vi "Grab Frame.vi"(5 "Live?":bool, 7 "Grab frame?":bool, 8 "error in (no error)":errorcluster, 9 "Rigid Body":T1, 11 "Frame Grabber Data in":T4={"Camera Session"="", "Frame"=refnum, "AVI Refnum"=refnum, "Codecs"=[], "Frame number"=0, "Tracking File Refnum"=refnum, "Tick Count"=0, "Probe Object"=refnum, "Playback Probe Data"=[], "Rigid Body"={"Position"={"x (mm)"=0.0, "y (mm)"=0.0, "z (mm)"=0.0}, "Orientation"={"Pitch (rad)"=0.0, "Yaw (rad)"=0.0, "Roll (rad)"=0.0}, "Quaternion"={"qx"=0.0, "qy"=0.0, "qz"=0.0, "qw"=0.0}, "Tracked?"=FALSE}, "Total no frames playback"=0, "Video FPS"=0.0, "Camera connected?"=FALSE, "Scene"=refnum, "Cropped Frame"=refnum, "Tracker FPS"=0.0, "Crop ROI"=[], "Presentation Values"=[], "Elapsed time (ms)"=0, "Camera frames playback"=0, "Refnums"={"Live Refnum"=refnum, "Record Refnum"=refnum, "Recording Settings Refnum"=refnum, "Playback Refnum"=refnum, "Frame Slider Refnum"=refnum, "Pause Refnum"=refnum, "Home Refnum"=refnum, "Crop Refnum"=refnum, "Clear Crop Refnum"=refnum, "stop refnum"=refnum, "Playback Rate Refnum"=refnum, "Operator Settings Refnums"=refnum, "Presentation Refnum"=refnum, "Gestation Refnum"=refnum, "Connection Settings Refnum"=refnum, "Crop Time Frame Slider Refnum"=refnum, "Cancel Save Refnum"=refnum, "Reverse Playback Refnum"=refnum}, "Dimensions"={"Probe Dimensions"={"Probe Width"=0.0, "Probe Depth"=1.0, "Probe Height"=0.0}, "Room Dimensions"={"Room Width"=0.0, "Room Depth"=0.0, "Room Height"=0.0}}, "Playback Data As Strings"=[], "Cropped Tracking File Refnum"=refnum, "Cropped AVI Refnum"=refnum, "Header"=[], "Total euclidian distance"=0.0}) -> (0 "error out":errorcluster, 1 "Elapsed time (ms)":u32, 2 "Frame":T6, 3 "Frame Grabber Data out":T4={"Camera Session"="", "Frame"=refnum, "AVI Refnum"=refnum, "Codecs"=[], "Frame number"=0, "Tracking File Refnum"=refnum, "Tick Count"=0, "Probe Object"=refnum, "Playback Probe Data"=[], "Rigid Body"={"Position"={"x (mm)"=0.0, "y (mm)"=0.0, "z (mm)"=0.0}, "Orientation"={"Pitch (rad)"=0.0, "Yaw (rad)"=0.0, "Roll (rad)"=0.0}, "Quaternion"={"qx"=0.0, "qy"=0.0, "qz"=0.0, "qw"=0.0}, "Tracked?"=FALSE}, "Total no frames playback"=0, "Video FPS"=0.0, "Camera connected?"=FALSE, "Scene"=refnum, "Cropped Frame"=refnum, "Tracker FPS"=0.0, "Crop ROI"=[], "Presentation Values"=[], "Elapsed time (ms)"=0, "Camera frames playback"=0, "Refnums"={"Live Refnum"=refnum, "Record Refnum"=refnum, "Recording Settings Refnum"=refnum, "Playback Refnum"=refnum, "Frame Slider Refnum"=refnum, "Pause Refnum"=refnum, "Home Refnum"=refnum, "Crop Refnum"=refnum, "Clear Crop Refnum"=refnum, "stop refnum"=refnum, "Playback Rate Refnum"=refnum, "Operator Settings Refnums"=refnum, "Presentation Refnum"=refnum, "Gestation Refnum"=refnum, "Connection Settings Refnum"=refnum, "Crop Time Frame Slider Refnum"=refnum, "Cancel Save Refnum"=refnum, "Reverse Playback Refnum"=refnum}, "Dimensions"={"Probe Dimensions"={"Probe Width"=0.0, "Probe Depth"=1.0, "Probe Height"=0.0}, "Room Dimensions"={"Room Width"=0.0, "Room Depth"=0.0, "Room Height"=0.0}}, "Playback Data As Strings"=[], "Cropped Tracking File Refnum"=refnum, "Cropped AVI Refnum"=refnum, "Header"=[], "Total euclidian distance"=0.0})   [LabVIEW 2017]
uses:
  <vilib>/vision/Image Controls.llb/IMAQ Image.ctl
  Controls/Frame Grabber Data.ctl
  <vilib>/userdefined/High Color/IMAQdx.ctl
  <vilib>/vision/Avi.llb/IMAQ AVI2 Refnum.ctl
  Controls/Rigid Body Info.ctl
  Controls/Position.ctl
  Controls/Orientation.ctl
  Controls/Refnums.ctl
  Controls/Recording Settings.ctl
  Controls/Operator Settings.ctl
  Controls/Operator.ctl
  Controls/Dimensions.ctl
  Controls/Room Dimensions.ctl
  <vilib>/vision/driver/NI_Vision_Acquisition_Software.lvlib
  <vilib>/vision/NI_Vision_Development_Module.lvlib
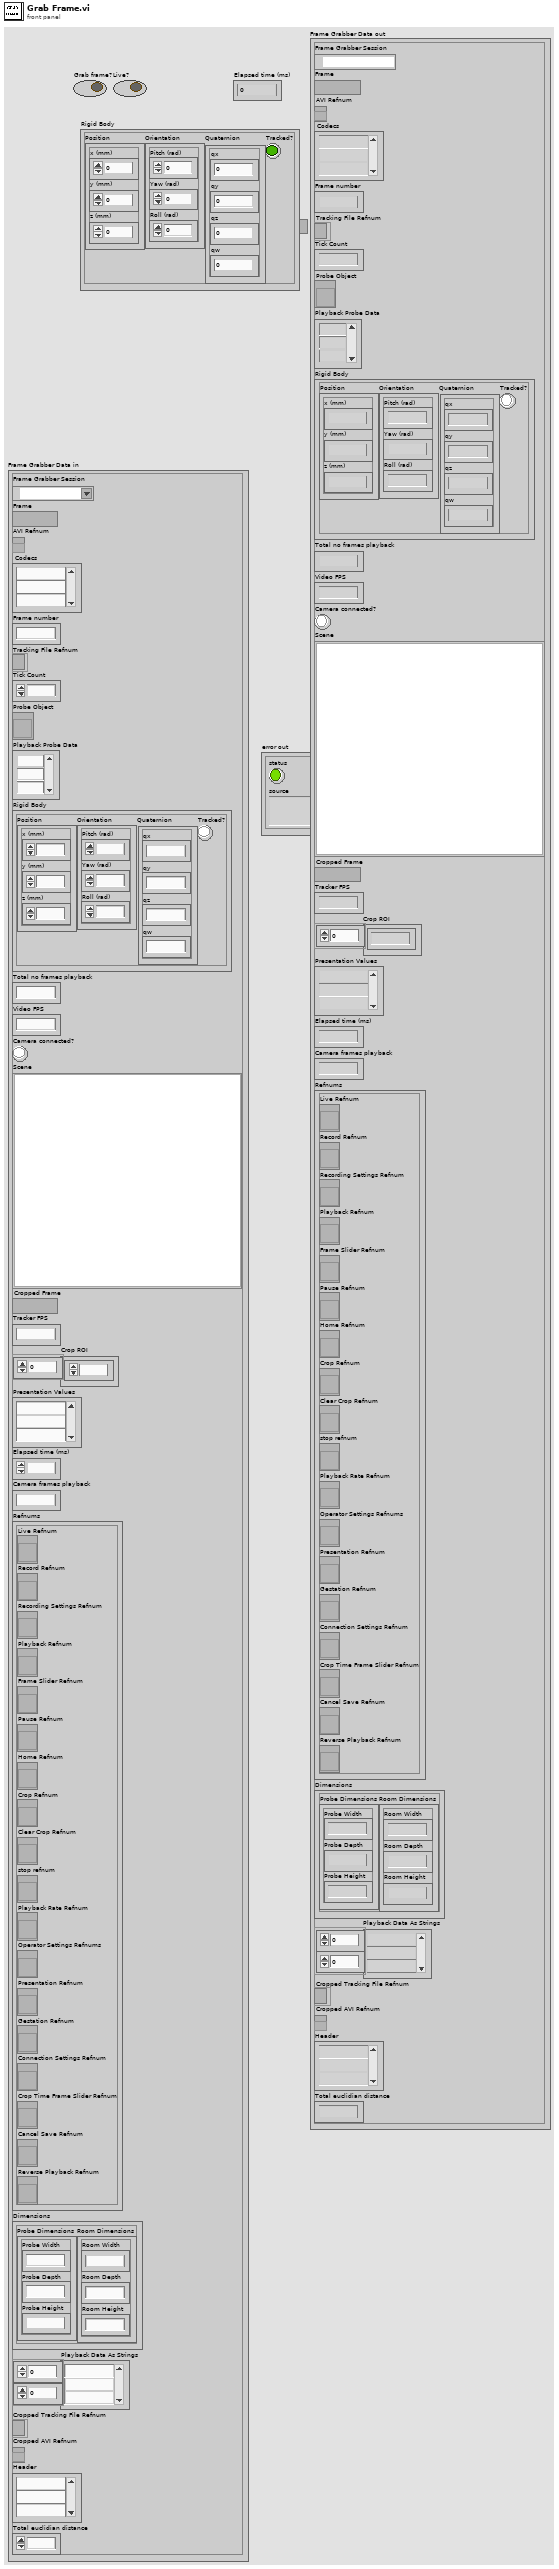
[diagram p1: front panel]
types:
  T1 = typedef "Rigid Body Info.ctl" = cluster{"Position":T2, "Orientation":T3, "Quaternion":cluster{"qx":sgl, "qy":sgl, "qz":sgl, "qw":sgl}, "Tracked?":bool}
  T2 = typedef "Position.ctl" = cluster{"x (mm)":sgl, "y (mm)":sgl, "z (mm)":sgl}
  T3 = typedef "Orientation.ctl" = cluster{"Pitch (rad)":sgl, "Yaw (rad)":sgl, "Roll (rad)":sgl}
  T4 = typedef "Frame Grabber Data.ctl" = cluster{"Camera Session":T5, "Frame":T6, "AVI Refnum":T7, "Codecs":string[], "Frame number":u32, "Tracking File Refnum":refnum<file>, "Tick Count":u32, "Probe Object":refnum<vi>, "Playback Probe Data":dbl[][], "Rigid Body":T1, "Total no frames playback":i32, "Video FPS":dbl, "Camera connected?":bool, "Scene":refnum<vi>, "Cropped Frame":T6, "Tracker FPS":dbl, "Crop ROI":i32[], "Presentation Values":string[], "Elapsed time (ms)":u32, "Camera frames playback":u32, "Refnums":T8, "Dimensions":T9, "Playback Data As Strings":string[][], "Cropped Tracking File Refnum":refnum<file>, "Cropped AVI Refnum":T7, "Header":string[], "Total euclidian distance":dbl}
  T5 = typedef "IMAQdx.ctl" = refnum<k21>
  T6 = typedef "IMAQ Image.ctl" = refnum<image>
  T7 = typedef "IMAQ AVI2 Refnum.ctl" = refnum<k20>
  T8 = typedef "Refnums.ctl" = cluster{"Live Refnum":refnum<vi>, "Record Refnum":refnum<vi>, "Recording Settings Refnum":refnum<vi>, "Playback Refnum":refnum<vi>, "Frame Slider Refnum":refnum<vi>, "Pause Refnum":refnum<vi>, "Home Refnum":refnum<vi>, "Crop Refnum":refnum<vi>, "Clear Crop Refnum":refnum<vi>, "stop refnum":refnum<vi>, "Playback Rate Refnum":refnum<vi>, "Operator Settings Refnums":refnum<vi>, "Presentation Refnum":refnum<vi>, "Gestation Refnum":refnum<vi>, "Connection Settings Refnum":refnum<vi>, "Crop Time Frame Slider Refnum":refnum<vi>, "Cancel Save Refnum":refnum<vi>, "Reverse Playback Refnum":refnum<vi>}
  T9 = typedef "Dimensions.ctl" = cluster{"Probe Dimensions":cluster{"Probe Width":sgl, "Probe Depth":sgl, "Probe Height":sgl}, "Room Dimensions":T10}
  T10 = typedef "Room Dimensions.ctl" = cluster{"Room Width":dbl, "Room Depth":dbl, "Room Height":dbl}
  T11 = typedef "Recording Settings.ctl" = cluster{"Folder to Save Recording":path, "Recording Name":string, "Video FPS":u32, "Codec":u16, "Tracker FPS":dbl}
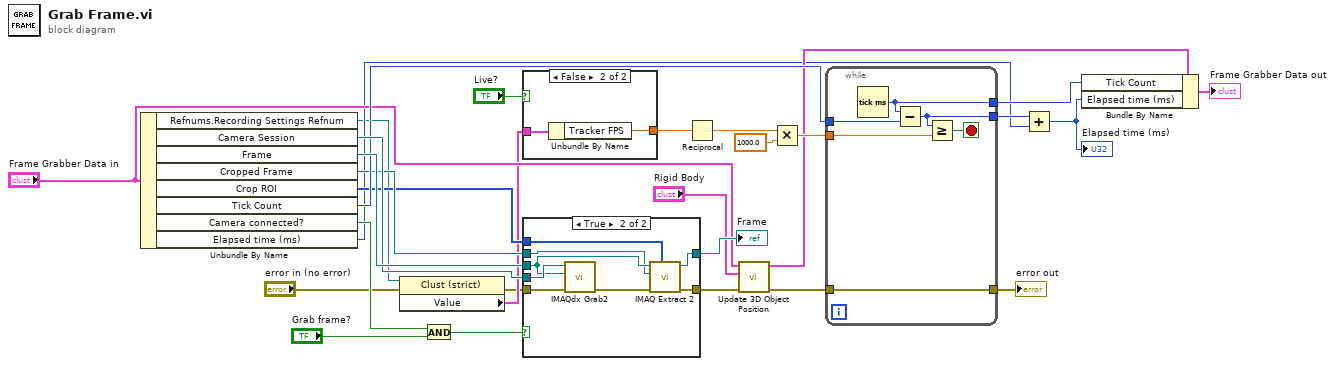
[diagram p0: block diagram]
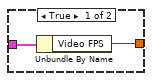
[diagram p2: hidden frame]
diagram:
  n1 = Unbundle By Name("Frame Grabber Data in") -> ("Refnums.Recording Settings Refnum"=w4:refnum<vi>, "Camera Session"=w24:T5, "Frame"=w25:T6, "Cropped Frame"=w12:T6, "Crop ROI"=w11:i32[], "Tick Count"=w20:u32, "Camera connected?"=w13:bool, "Elapsed time (ms)"=w5:u32)
  n2 = property class="Clust (strict)"(reference=w4, error in="error in (no error)") -> (error out=w1:errorcluster, "Value"=w3:T11)  [unwired: 1 out]
  n3 = And(x=w13, y="Grab frame?") -> (x .and. y?=w10:bool)
  n4 = case shown="False" "Live?" {
    tunnel: w3 -> [w31 w33]
    tunnel: [w30 w32] -> w27
    frame True {
      n5 = Unbundle By Name(w31) -> ("Video FPS"=w30:u32)
    }
    frame False {
      n6 = Unbundle By Name(w33) -> ("Tracker FPS"=w32:dbl)
    }
  }
  n7 = case shown="True" w10 {
    tunnel: w25 -> [_ w40]
    tunnel: w24 -> [_ w43]
    tunnel: [w34 w38] -> w23
    tunnel: w1 -> [w35 w42]
    tunnel: [w35 w37] -> w18
    tunnel: w12 -> [w34 w39]
    tunnel: w11 -> [_ w41]
    frame False {
    }
    frame True {
      n8 = call <vilib>:"IMAQdx Grab2.vi"("error in"=w42, "Image In"=w40, "Session In"=w43) -> ("error out"=w36:errorcluster)  [unwired: 5 in, 3 out]
      n9 = call "IMAQ Extract 2"("Optional Rectangle"=w41, "error in (no error)"=w36, "Image Dst"=w39, "Image Src"=w40) -> ("error out"=w37:errorcluster, "Image Dst Out"=w38:T6)  [unwired: 6 in]
    }
  }
  "Frame" <- w23
  n10 = Reciprocal(x=w27) -> (1/x=w26:dbl)
  n11 = call "Update 3D Object Position.vi"("error in (no error)"=w18, "New Rigid Body Position"="Rigid Body", "Frame Grabber Data in"="Frame Grabber Data in") -> ("error out"=w17:errorcluster, "Frame Grabber Data out"=w14:T4)  [unwired: 7 in]
  n12 = Multiply(x=w26, y=1000.0) -> (x*y=w29:dbl)
  n13 = while {
    tunnel: [w49] -> w22
    tunnel: w29 -> [w47]
    tunnel: w20 -> [w46]
    tunnel: w17 -> [w45]
    tunnel: [w45] -> w19
    tunnel: [w44] -> w7
    stop <- w48 stop-if-true
    n14 = Tick Count (ms)() -> (millisecond timer value=w49:u32)
    n15 = Subtract(x=w49, y=w46) -> (x-y=w44:u32)
    n16 = Greater Or Equal?(x=w44, y=w47) -> (x >= y?=w48:bool)
  }
  "error out" <- w19
  n17 = Add(x=w7, y=w5) -> (x+y=w6:u32)
  "Elapsed time (ms)" <- w6
  n18 = Bundle By Name(cluster=w14, "Tick Count"=w22, "Elapsed time (ms)"=w6) -> (→"Frame Grabber Data out":T4)
